vi "Washer HCC Tool.vi"() -> ()   [LabVIEW 2009]
panel:
  in  "Backup Batch File":path=path "c:/Program Files/GE/Washer HCC/robocopy_update.bat"
  out "COM Port":string
  in  "Station":u16(ring) items=["1", "2", "3", "4", "5", "6", "7", "8", "9", "10", "11", "12", "13", "14", "15", "16", "17", "18", "19", "20"]
  in  "Row":u16(ring) items=["A", "B", "C", "D", "E", "F", "G", "H", "I", "J", "M", "N", "S"]
  in  "Save Now":bool
  out "Filename":string
  out "Min to AutoSave":dbl format="%#_3g"
  in  "AutoSave Period(min)":dbl=60.0
  in  "Serial":string="E15"
  in  "Unit":string="asssdf"
  out "date/time string":string
  in  "Station Com Unit Serial Array":string[][](array[string])
  in  "Clipboard":bool
  in  "OK":bool
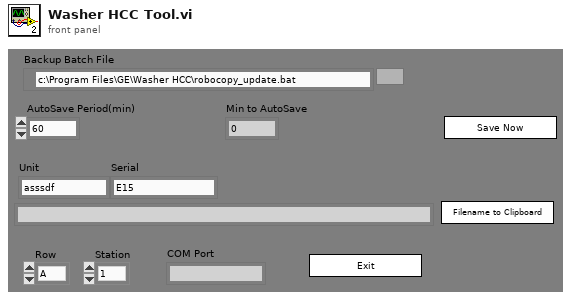
[diagram p1: front panel]
types:
  T1 = enum32{"invalid app kind", "Development System", "Run Time System", "Student Edition", "Embedded LabVIEW", "Evaluation", "Custom"}
  T2 = enum32{"Invalid", "Standard", "Closed", "Hidden", "Minimized", "Maximized"}
  T3 = cluster{"Core":cluster{"Current VI Reference":refnum<vi>, "Close Panel on Exit?":bool}, "Your Boolean data":bool, "Station Com Unit Serial Array":string[][], "Elapsed Time (sec)":dbl}
  T4 = cluster{"Current VI Reference":refnum<vi>, "Close Panel on Exit?":bool}
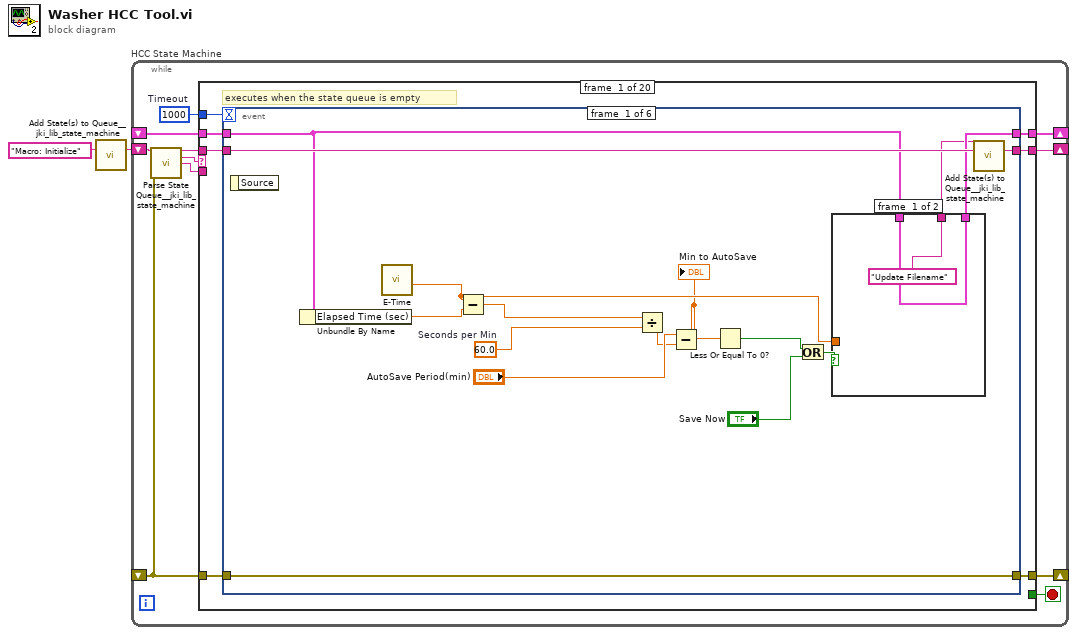
[diagram p0: block diagram]
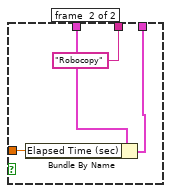
[diagram p2: hidden frame]
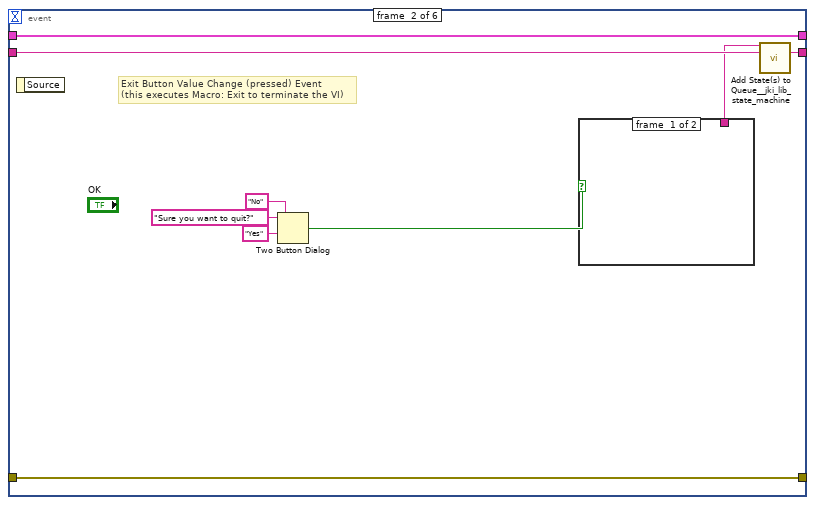
[diagram p3: hidden frame]
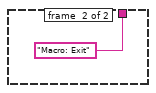
[diagram p4: hidden frame]
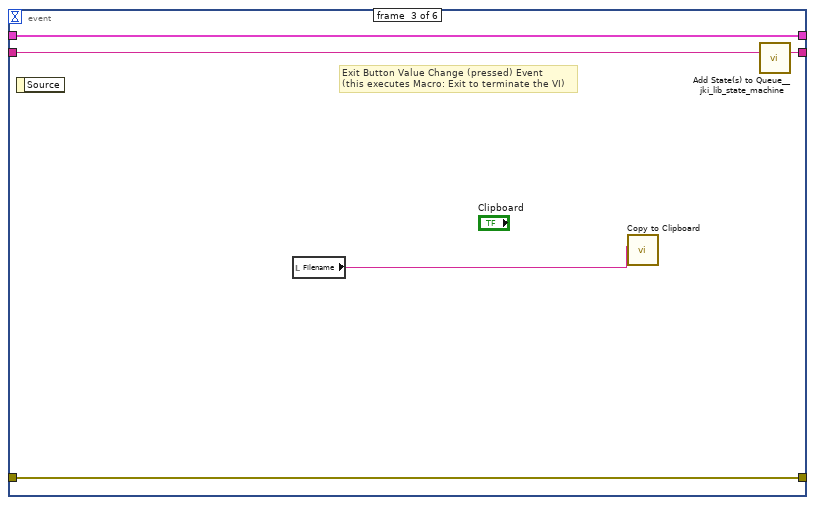
[diagram p5: hidden frame]
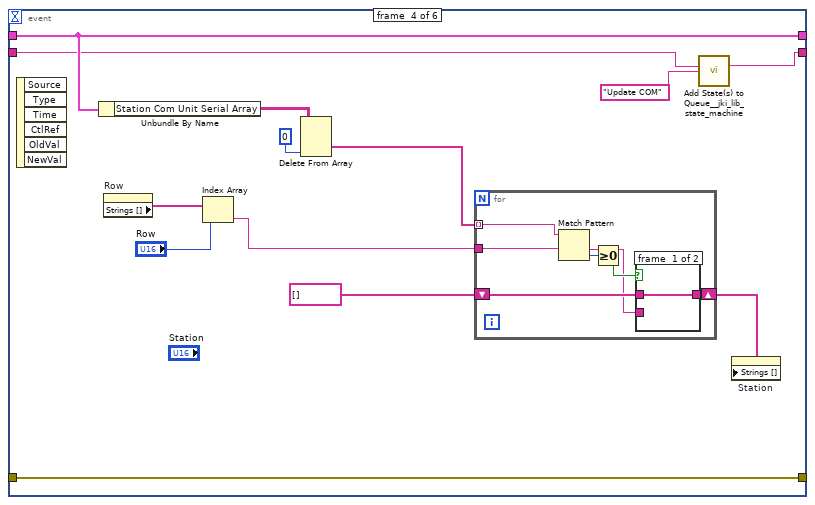
[diagram p6: hidden frame]
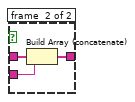
[diagram p7: hidden frame]
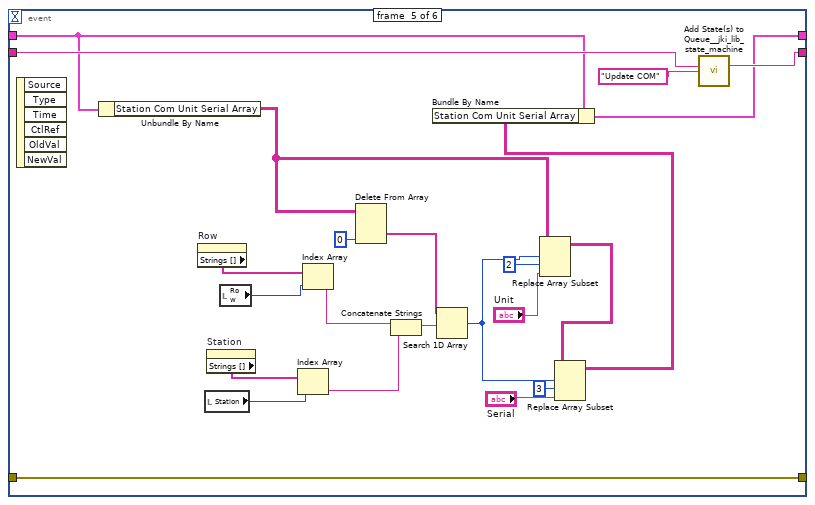
[diagram p8: hidden frame]
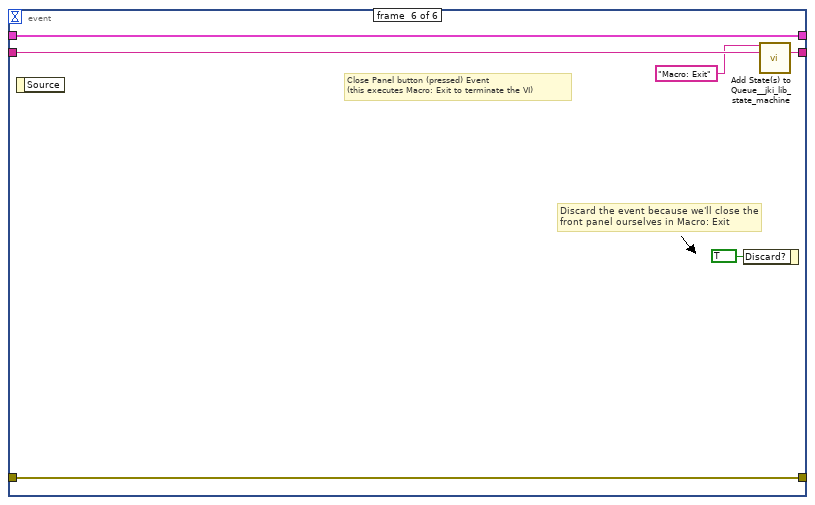
[diagram p9: hidden frame]
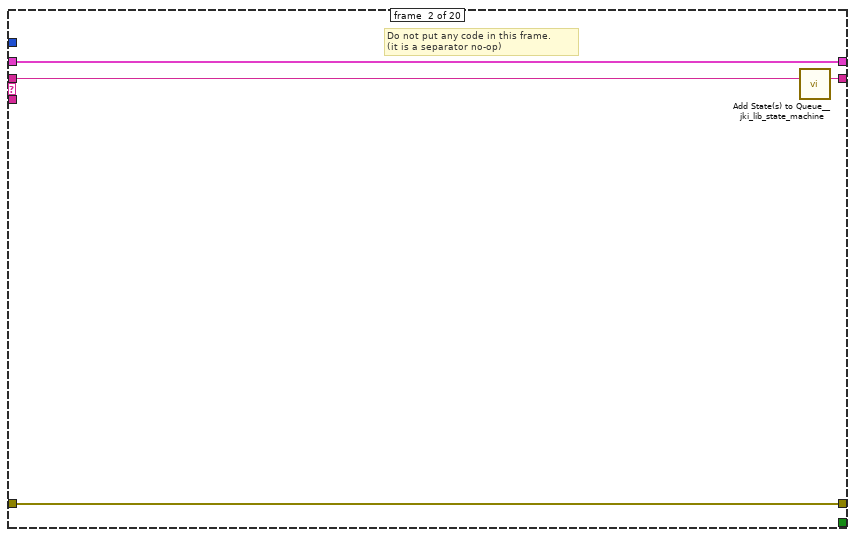
[diagram p10: hidden frame]
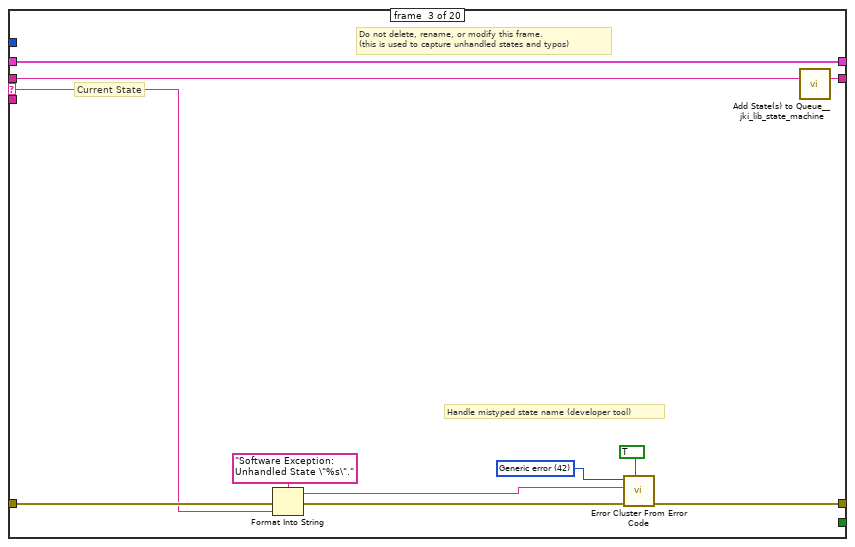
[diagram p11: hidden frame]
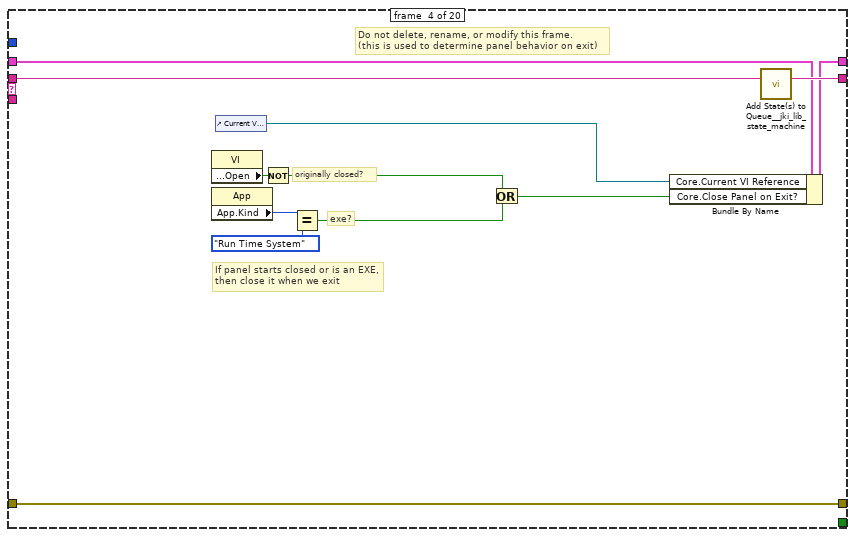
[diagram p12: hidden frame]
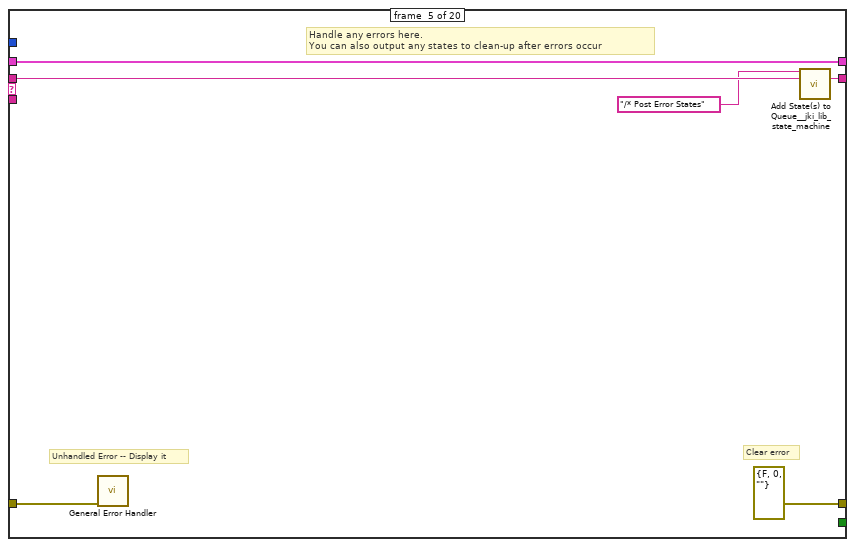
[diagram p13: hidden frame]
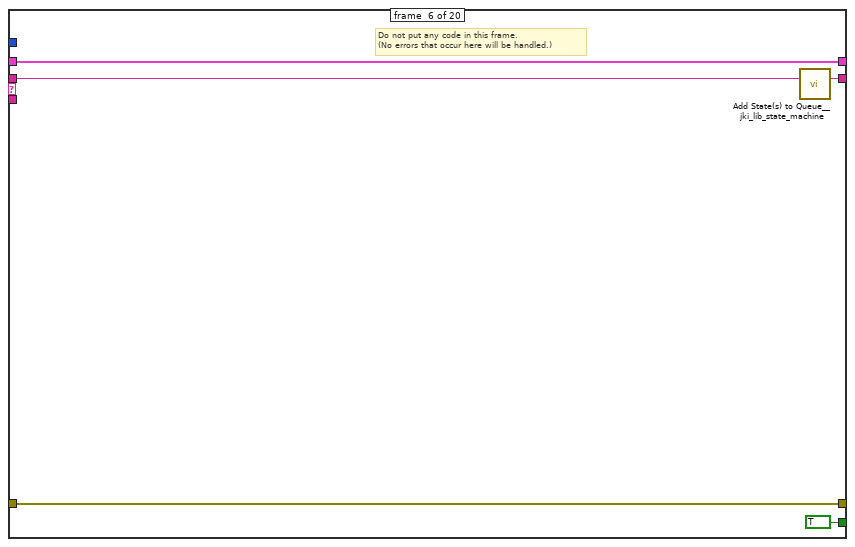
[diagram p14: hidden frame]
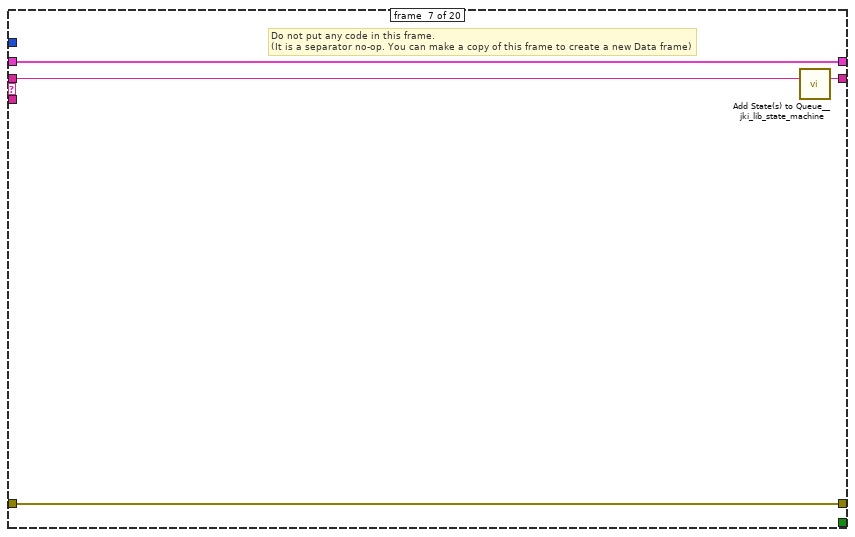
[diagram p15: hidden frame]
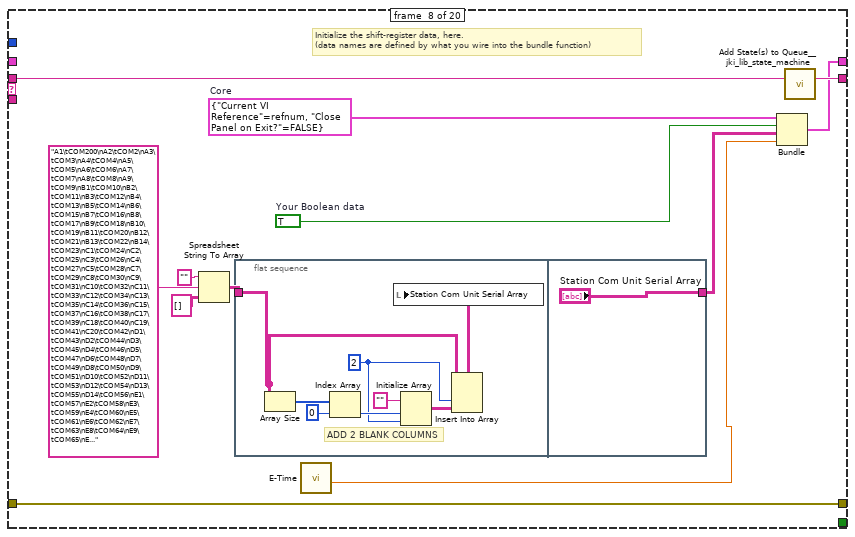
[diagram p16: hidden frame]
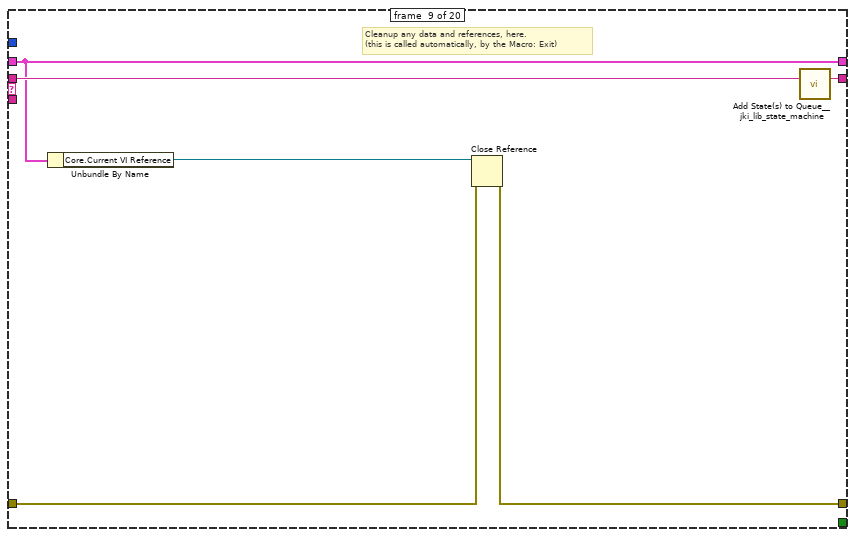
[diagram p17: hidden frame]
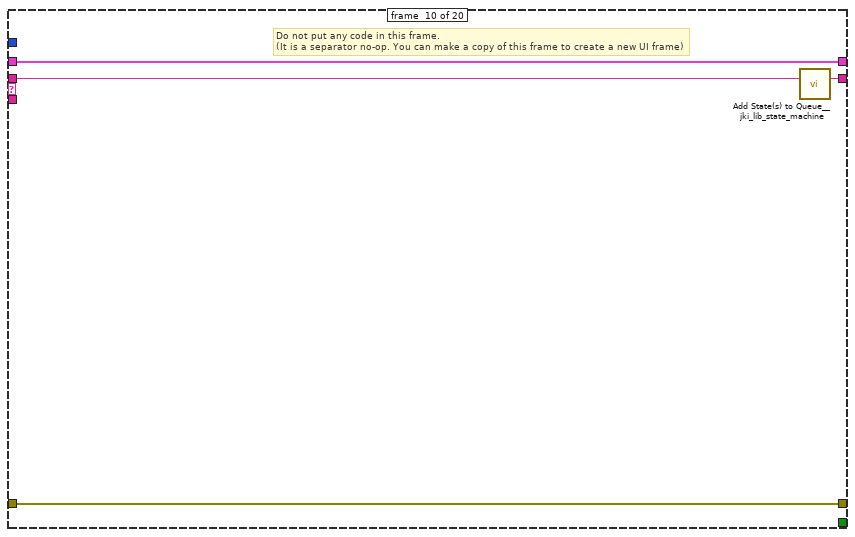
[diagram p18: hidden frame]
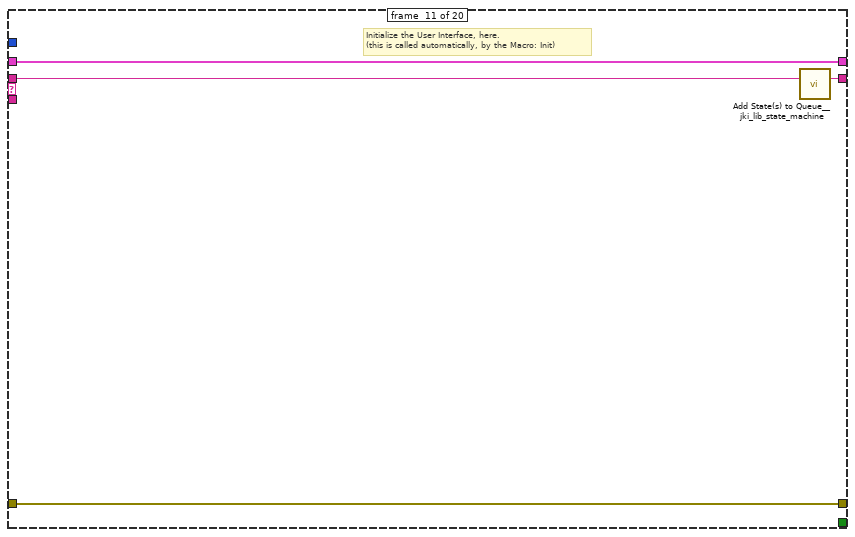
[diagram p19: hidden frame]
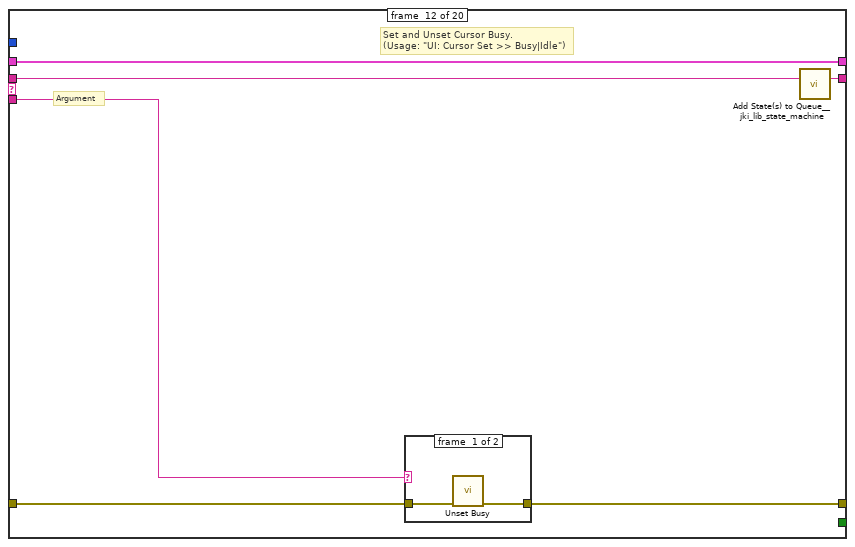
[diagram p20: hidden frame]
diagram:
  n1 = call <vilib>:"Add State(s) to Queue__jki_lib_state_machine.vi"("State(s) in (\"\")"="Macro: Initialize") -> ("States Out"=w2:string)  [unwired: 14 in]
  n2 = while "HCC State Machine" {
    shift-right: [w6] -> _
    shift-left: _ -> [w5]
    shift-right: [w9] -> _
    shift-left: _ -> [w3]
    shift-right: [w8] -> _
    shift-left: w2 -> [w10]
    stop <- w7 stop-if-true
    w4 = 1000  # Timeout
    n3 = call <vilib>:"Parse State Queue__jki_lib_state_machine.vi"("State Queue"=w10, "Error In (no error)"=w3) -> ("Remaining States"=w12:string, "Current State"=w13:string, "Arguments"=w11:string)  [unwired: 11 in]
    n4 = case shown="\"Data: Cleanup\"" w13 {
      selector: w13 -> [_ _ w115 _ _ _ _ _ _ _ _ _ _ _ _ _ _ _ _ _]
      tunnel: w12 -> [w20 w114 w119 w137 w143 w148 w152 w164 w179 w183 w187 w193 w204 w230 w235 w245 w249 w269 w276 w300]
      tunnel: w11 -> [_ _ _ _ _ _ _ _ _ _ _ w188 w198 _ _ _ _ _ _ _]
      tunnel: w5 -> [w18 w111 w117 w128 w140 w146 w149 _ w174 w180 w185 w191 w200 w227 w232 w242 w246 w266 w274 w297]
      tunnel: [w17 w112 w121 w134 errorcluster {"status"=FALSE, "code"=0, "source"=""} ("error out") w145 w150 w161 w175 w181 w184 w189 w201 w228 w233 w243 w247 w267 w272 w298] -> w9
      tunnel: w3 -> [w16 w112 w120 w134 w139 w145 w150 w161 w176 w181 w184 w190 w202 w228 w233 w243 w247 w267 w273 w298]
      tunnel: [w19 w113 w118 w136 w142 w147 w151 w163 w178 w182 w186 w192 w203 w229 w234 w244 w248 w268 w275 w299] -> w8
      tunnel: [_ _ _ _ _ TRUE _ _ _ _ _ _ _ _ _ _ _ _ _ _] -> w7
      tunnel: [w15 w111 w117 w135 w140 w146 w149 w162 w174 w180 w185 w191 w200 w227 w232 w242 w246 w266 w274 w297] -> w6
      tunnel: w4 -> [w14 _ _ _ _ _ _ _ _ _ _ _ _ _ _ _ _ _ _ _]
      frame #0 {
        # "executes when the state queue is empty"
        n5 = event shown="[4] \"Unit\", \"Serial\": Value Change" {
          selector: _ -> [_ _ _ _ _ _]
          dyn-events: _ -> [_ _ _ _ _ _]
          timeout: w14 -> [_ _ _ _ _ _]
          tunnel: w20 -> [w36 w51 w57 w60 w103 w110]
          tunnel: [w35 w50 w56 w59 w102 w109] -> w19
          tunnel: w18 -> [w28 w48 w54 w70 w90 w107]
          tunnel: [w34 w49 w55 w69 w104 w108] -> w17
          tunnel: w16 -> [w34 w49 w55 w69 w104 w108]
          tunnel: [w27 w48 w54 w70 w91 w107] -> w15
          event #0 {
            w31 = 60.0  # Seconds per Min
            n6 = event-data() -> ()  [unwired: 1 in, 1 out]
            n7 = Unbundle By Name(w28) -> ("Elapsed Time (sec)"=w33:dbl)
            n8 = call "E-Time.vi"() -> ("Elapsed Time (sec)"=w26:dbl)  [unwired: 9 in, 2 out]
            n9 = Subtract(x=w26, y=w33) -> (x-y=w32:dbl)
            n10 = Divide(x=w32, y=w31) -> (x/y=w22:dbl)
            n11 = Subtract(x="AutoSave Period(min)", y=w22) -> (x-y=w24:dbl)
            "Min to AutoSave" <- w24
            n12 = Less Or Equal To 0?(x=w24) -> (x <= 0?=w30:bool)
            n13 = Or(x=w30, y="Save Now") -> (x .or. y?=w29:bool)
            n14 = case shown="False" w29 {
              tunnel: w28 -> [w38 w41]
              tunnel: [w38 w42] -> w27
              tunnel: w26 -> [_ w40]
              tunnel: ["Update Filename" ("State(s) in Front (\"\")") "Robocopy" ("State(s) in Front (\"\")")] -> w25
              frame #0 {
              }
              frame #1 {
                n15 = Bundle By Name(cluster=w41, "Elapsed Time (sec)"=w40) -> (w42:T3)
              }
            }
            n16 = call <vilib>:"Add State(s) to Queue__jki_lib_state_machine.vi"("State(s) in Front (\"\")"=w25, "State(s) in (\"\")"=w36) -> ("States Out"=w35:string)  [unwired: 13 in]
          }
          event #1 {
            # "Exit Button Value Change (pressed) Event\n(this executes Macro: Exit to terminate the VI)"
            n17 = event-data() -> ()  [unwired: 1 in, 1 out]
            n18 = Two Button Dialog(message="Sure you want to quit?", 1:"No" ("F button name (\"Cancel\")"), 2:"Yes" ("T button name (\"OK\")")) -> (T button?=w43:bool)
            n19 = case shown="True" w43 {
              tunnel: [_ "Macro: Exit"] -> w47
              frame #0 {
              }
              frame #1 {
              }
            }
            n20 = call <vilib>:"Add State(s) to Queue__jki_lib_state_machine.vi"("State(s) in Front (\"\")"=w47, "State(s) in (\"\")"=w51) -> ("States Out"=w50:string)  [unwired: 13 in]
          }
          event #2 {
            # "Exit Button Value Change (pressed) Event\n(this executes Macro: Exit to terminate the VI)"
            n21 = event-data() -> ()  [unwired: 1 in, 1 out]
            n22 = local read "Filename"() -> (w53:string)
            n23 = call "Copy to Clipboard.vi"("Text"=w53) -> ()  [unwired: 11 in]
            n24 = call <vilib>:"Add State(s) to Queue__jki_lib_state_machine.vi"("State(s) in (\"\")"=w57) -> ("States Out"=w56:string)  [unwired: 14 in]
          }
          event #3 {
            n25 = event-data() -> ()  [unwired: 1 in, 6 out]
            n26 = Unbundle By Name(w70) -> ("Station Com Unit Serial Array"=w66:string[][])
            n27 = property on="Row" class="Ring (strict)"() -> ("Strings []"=w68:string[])  [unwired: 2 in, 2 out]
            n28 = Index Array(array=w68, index="Row") -> (element=w63:string)
            n29 = Delete From Array(array=w66, index (col)=0 ("length")) -> (deleted portion=w65:string[])  [unwired: 2 in, 1 out]
            n30 = for {
              tunnel: w65 -> [w77] mode=indexing
              tunnel: w63 -> [w76]
              shift-right: [w73] -> w61
              shift-left: string[] [] ("deleted portion") -> [w72]
              n31 = Match Pattern(string=w77, regular expression=w76) -> (after substring=w71:string, offset past match=w75:i32)  [unwired: 1 in, 2 out]
              n32 = Greater Or Equal To 0?(x=w75) -> (x >= 0?=w74:bool)
              n33 = case shown="True" w74 {
                tunnel: [w78 w80] -> w73
                tunnel: w72 -> [w78 w81]
                tunnel: w71 -> [_ w79]
                frame #0 {
                }
                frame #1 {
                  n34 = Build Array (concatenate)(w81, w79) -> (w80:string[])
                }
              }
            }
            n35 = call <vilib>:"Add State(s) to Queue__jki_lib_state_machine.vi"("State(s) in (\"\")"=w60, "State(s) at Back (\"\")"="Update COM" ("State(s) at Back (\"\")")) -> ("States Out"=w59:string)  [unwired: 13 in]
            n36 = property on="Station" class="Ring (strict)"("Strings []"=w61) -> ()  [unwired: 2 in, 2 out]
          }
          event #4 {
            n37 = event-data() -> ()  [unwired: 1 in, 6 out]
            n38 = Unbundle By Name(w90) -> ("Station Com Unit Serial Array"=w89:string[][])
            n39 = property on="Row" class="Ring (strict)"() -> ("Strings []"=w100:string[])  [unwired: 2 in, 2 out]
            n40 = local read "Station"() -> (w97:u16)
            n41 = property on="Station" class="Ring (strict)"() -> ("Strings []"=w98:string[])  [unwired: 2 in, 2 out]
            n42 = local read "Row"() -> (w99:u16)
            n43 = Index Array(array=w98, index=w97) -> (element=w95:string)
            n44 = Index Array(array=w100, index=w99) -> (element=w96:string)
            n45 = Delete From Array(array=w89, index (col)=0 ("disabled index (col)")) -> (deleted portion=w92:string[])  [unwired: 2 in, 1 out]
            n46 = Concatenate Strings(w96, w95) -> (w94:string)
            n47 = Search 1D Array(1D array=w92, element=w94) -> (index of element=w84:i32)  [unwired: 1 in]
            n48 = Replace Array Subset(array=w89, new element="Unit", index (row)=w84, index (col)=2 ("disabled index (col)")) -> (w86:string[][])
            n49 = Replace Array Subset(array=w86, new element="Serial", index (row)=w84, index (col)=3 ("disabled index (col)")) -> (w82:string[][])
            n50 = Bundle By Name(cluster=w90, "Station Com Unit Serial Array"=w82) -> (w91:T3)
            n51 = call <vilib>:"Add State(s) to Queue__jki_lib_state_machine.vi"("State(s) in (\"\")"=w103, "State(s) at Back (\"\")"="Update COM" ("State(s) at Back (\"\")")) -> ("States Out"=w102:string)  [unwired: 13 in]
          }
          event #5 {
            # "Discard the event because we'll close the front panel ourselves in Macro: Exit"
            # "Close Panel button (pressed) Event\n(this executes Macro: Exit to terminate the VI)"
            n52 = event-data() -> ()  [unwired: 1 in, 1 out]
            n53 = event-data("Discard?"=TRUE) -> ()  [unwired: 1 in, 1 out]
            n54 = call <vilib>:"Add State(s) to Queue__jki_lib_state_machine.vi"("State(s) in Front (\"\")"="Macro: Exit", "State(s) in (\"\")"=w110) -> ("States Out"=w109:string)  [unwired: 13 in]
          }
        }
      }
      frame #1 {
        # "Do not put any code in this frame.\n(it is a separator no-op)"
        n55 = call <vilib>:"Add State(s) to Queue__jki_lib_state_machine.vi"("State(s) in (\"\")"=w114) -> ("States Out"=w113:string)  [unwired: 14 in]
      }
      frame #2 {
        w124 = 42 items=["No error", "Argument error", "Memory is full", "Out of zone", "End of file", "File already open", "Generic file I/O error", "File not found", "File permission error", "Disk is full", "Duplicate path", "Too many files open", "System feature not enabled", "Resource file not found", "Cannot add resource", "Resource not found", "Image not found", "Image memory error", "Pen does not exist", "Config type invalid", "Config token not found", "Config parse error", "Config memory error", "Bad external code format", "Bad external code offset", "External code not present", "Null window", "Destroy window error", "Null menu", "Print aborted", "Bad print record", "Print driver error", "Windows error during printing", "Memory error during printing", "Print dialog error", "Generic print error", "Invalid device refnum", "Device not found", "Device parameter error", "Device unit error", "Cannot open device", "Device call aborted", "Generic error", "Cancelled by user", "Object ID too low", "Object ID too high", "Object not in heap", "Unknown heap", "Unknown object (invalid DefProc)", "Unknown object (DefProc not in table)", "Message out of range", "Invalid (null) method", "Unknown message", "Manager call not supported", "Bad address", "Network operation in progress", "Network operation timed out", "Connection is busy", "Network attribute not supported", "Network error", "Address in use", "System out of memory", "Connection aborted", "Connection refused", "Not connected", "Already connected", "Connection closed", "Initialization error (interapplication manager)", "Bad occurrence", "Wait on unbound occurrence handler", "Occurrence queue overflow", "Datalog type conflict", "Unused", "Unrecognized type (interapplication manager)", "Memory corrupt", "Failed to make temporary DLL", "Old CIN version", "Drag socket not found", "Failed to load drop-object", "Failed to register OLE object", "Failed to release OLE object", "Format specifier type mismatch", "Unknown format specifier", "Too few format specifiers", "Too many format specifiers", "Scan failed", "Newer CIN version", "Error converting to variant", "Runtime menu error", "Password tampered", "Variant attribute not found", "Incompatible variant data type", "Event data is not available", "Event Store is not present", "Occurrence is not found", "Event Queue is not created", "Event info is not available", "Refnum passed is NULL", "Error retrieving Class GUID", "Error retrieving CoClass GUID", "Error retrieving TypeLib GUID.", "Bad built application magic bytes.", "Specific driver is different from the specific driver associated with the Logical Name.", "There is no session opened to the class driver.", "Max Error", "MAX - Error with config objects", "MAX - Error loading configuration", "MAX - Group not supported"]
        # "Current State"
        # "Do not delete, rename, or modify this frame.\n(this is used to capture unhandled states and typos)"
        # "Handle mistyped state name (developer tool)"
        n56 = Format Into String(format string="Software Exception: Unhandled State \"%s\"." ("message"), error in=w120, w115) -> (resulting string=w123:string, error out=w122:errorcluster)  [unwired: 1 in]
        n57 = call <vilib>:"Error Cluster From Error Code.vi"("show call chain? (False)"=TRUE, "error in (no error)"=w122, "error message (\"\")"=w123, "error code (0)"=w124) -> ("error out"=w121:errorcluster)  [unwired: 5 in]
        n58 = call <vilib>:"Add State(s) to Queue__jki_lib_state_machine.vi"("State(s) in (\"\")"=w119) -> ("States Out"=w118:string)  [unwired: 14 in]
      }
      frame #3 {
        # "Do not delete, rename, or modify this frame.\n(this is used to determine panel behavior on exit)"
        # "originally closed?"
        # "exe?"
        # "If panel starts closed or is an EXE, then close it when we exit"
        n59 = property class="VI"() -> ("Front Panel.Open"=w133:bool)  [unwired: 2 in, 2 out]
        n60 = property class="App"() -> ("App.Kind"=w132:T1)  [unwired: 2 in, 2 out]
        n61 = control-ref of="Current VI Reference"() -> (w126:refnum<vi>)
        n62 = Not(x=w133) -> (.not. x?=w130:bool)
        n63 = Equal?(x=w132, y=T1."Run Time System" ("Application:Kind")) -> (x = y?=w129:bool)
        n64 = Or(x=w130, y=w129) -> (x .or. y?=w127:bool)
        n65 = Bundle By Name(cluster=w128, "Core.Current VI Reference"=w126, "Core.Close Panel on Exit?"=w127) -> (w135:T3)
        n66 = call <vilib>:"Add State(s) to Queue__jki_lib_state_machine.vi"("State(s) in (\"\")"=w137) -> ("States Out"=w136:string)  [unwired: 14 in]
      }
      frame #4 {
        # "Unhandled Error -- Display it"
        # "Handle any errors here.\nYou can also output any states to clean-up after errors occur"
        # "Clear error"
        n67 = call <vilib>:"General Error Handler.vi"("error in (no error)"=w139) -> ()  [unwired: 10 in, 5 out]
        n68 = call <vilib>:"Add State(s) to Queue__jki_lib_state_machine.vi"("State(s) in Front (\"\")"="/* Post Error States", "State(s) in (\"\")"=w143) -> ("States Out"=w142:string)  [unwired: 13 in]
      }
      frame #5 {
        # "Do not put any code in this frame.\n(No errors that occur here will be handled.)"
        n69 = call <vilib>:"Add State(s) to Queue__jki_lib_state_machine.vi"("State(s) in (\"\")"=w148) -> ("States Out"=w147:string)  [unwired: 14 in]
      }
      frame #6 {
        # "Do not put any code in this frame.\n(It is a separator no-op. You can make a copy of this frame to create a new Data frame)"
        n70 = call <vilib>:"Add State(s) to Queue__jki_lib_state_machine.vi"("State(s) in (\"\")"=w152) -> ("States Out"=w151:string)  [unwired: 14 in]
      }
      frame #7 {
        w159 = T4 {"Current VI Reference"=refnum, "Close Panel on Exit?"=FALSE}  # Core
        w160 = TRUE  # Your Boolean data
        # "Initialize the shift-register data, here.\n(data names are defined by what you wire into the bundle function)"
        n71 = Spreadsheet String To Array(format string="", spreadsheet string="A1\tCOM200\nA2\tCOM2\nA3\tCOM3\nA4\tCOM4\nA5\tCOM5\nA6\tCOM6\nA7\tCOM7\nA8\tCOM8\nA9\tCOM9\nB1\tCOM10\nB2\tCOM11\nB3\tCOM12\nB4\tCOM13\nB5\tCOM14\nB6\tCOM15\nB7\tCOM16\nB8\tCOM17\nB9\tCOM18\nB10\tCOM19\nB11\tCOM20\nB12\tCOM21\nB13\tCOM22\nB14\tCOM23\nC1\tCOM24\nC2\tCOM25\nC3\tCOM26\nC4\tCOM27\nC5\tCOM28\nC7\tCOM29\nC8\tCOM30\nC9\tCOM31\nC10\tCOM32\nC11\tCOM33\nC12\tCOM34\nC13\tCOM35\nC14\tCOM36\nC15\tCOM37\nC16\tCOM38\nC17\tCOM39\nC18\tCOM40\nC19\tCOM41\nC20\tCOM42\nD1\tCOM43\nD2\tCOM44\nD3\tCOM45\nD4\tCOM46\nD5\tCOM47\nD6\tCOM48\nD7\tCOM49\nD8\tCOM50\nD9\tCOM51\nD10\tCOM52\nD11\tCOM53\nD12\tCOM54\nD13\tCOM55\nD14\tCOM56\nE1\tCOM57\nE2\tCOM58\nE3\tCOM59\nE4\tCOM60\nE5\tCOM61\nE6\tCOM62\nE7\tCOM63\nE8\tCOM64\nE9\tCOM65\nE10\tCOM66\nE11\tCOM67\nE12\tCOM68\nE13\tCOM69\nE14\tCOM70\nE15\tCOM71\nE16\tCOM72\nE17\tCOM73\nE18\tCOM74\nE19\tCOM75\nE20\tCOM76\nF1\tCOM77\nF2\tCOM78\nF5\tCOM79\nF6\tCOM80\nF7\tCOM81\nF8\tCOM82\nF9\tCOM83\nF10\tCOM84\nF11\tCOM85\nF12\tCOM86\nF13\tCOM87\nG1\tCOM88\nG2\tCOM89\nG3\tCOM90\nG4\tCOM91\nG5\tCOM92\nG6\tCOM93\nG7\tCOM94\nG8\tCOM95\nG9\tCOM96\nG10\tCOM97\nG11\tCOM98\nG12\tCOM99\nG13\tCOM100\nG14\tCOM101\nH1\tCOM102\nH2\tCOM103\nH3\tCOM104\nH4\tCOM105\nH5\tCOM106\nH6\tCOM107\nH7\tCOM108\nH8\tCOM109\nH9\tCOM110\nH10\tCOM111\nI1\tCOM112\nI2\tCOM113\nI3\tCOM114\nI4\tCOM115\nI5\tCOM116\nI6\tCOM117\nI7\tCOM118\nI8\tCOM119\nI9\tCOM120\nI10\tCOM121\nI11\tCOM122\nI12\tCOM123\nM1\tCOM100\nM2\tCOM2\nM3\tCOM3\nM4\tCOM4\nM5\tCOM5\nM6\tCOM6\nM7\tCOM7\nM8\tCOM8\nM9\tCOM9\nM10\tCOM10\nM11\tCOM11\nM12\tCOM12\nM13\tCOM13\nM14\tCOM14\nM15\tCOM15\nM16\tCOM16\nM17\tCOM17\nM18\tCOM18\nM19\tCOM19\nM20\tCOM20\nN6\tCOM21\nN7\tCOM22\nN8\tCOM23\nN9\tCOM24\nN10\tCOM25\nN11\tCOM26\nN12\tCOM27\nN13\tCOM28\nS1\tCOM29\nS2\tCOM30\nS3\tCOM31\nS4\tCOM32\nS5\tCOM33\nS6\tCOM34\nS7\tCOM35\nS8\tCOM36\nS9\tCOM37\nS10\tCOM38\nS11\tCOM39\nS12\tCOM40\nS13\tCOM41\nS14\tCOM42\nS15\tCOM43\nS16\tCOM44\nS17\tCOM45\nS18\tCOM46\nS19\tCOM47\nS20\tCOM48\n", array type (2D Dbl)=string[][] []) -> (array=w154:string[][])  [unwired: 1 in]
        n72 = flat-sequence {
          tunnel: w154 -> [w166]
          tunnel: ["Station Com Unit Serial Array"] -> w157
          frame #0 {
            w169 = 2 ("index (row)")
            # "ADD 2 BLANK COLUMNS"
            n73 = Array Size(array=w166) -> (size(s)=w172:i32[])
            n74 = Index Array(array=w172, index=0) -> (element=w170:i32)
            n75 = Initialize Array("", w170, w169) -> (w167:string[][])
            n76 = Insert Into Array(array=w166, index (col)=w169, new element=w167) -> (w165:string[][])  [unwired: 1 in]
            n77 = local write "Station Com Unit Serial Array"(w165) -> ()
          }
          frame #1 {
          }
        }
        n78 = call "E-Time.vi"() -> ("Elapsed Time (sec)"=w153:dbl)  [unwired: 9 in, 2 out]
        n79 = Bundle("Core"=w159, "Your Boolean data"=w160, "Station Com Unit Serial Array"=w157, "Elapsed Time (sec)"=w153) -> (w162:T3)  [unwired: 1 in]
        n80 = call <vilib>:"Add State(s) to Queue__jki_lib_state_machine.vi"("State(s) in (\"\")"=w164) -> ("States Out"=w163:string)  [unwired: 14 in]
      }
      frame #8 {
        # "Cleanup any data and references, here.\n(this is called automatically, by the Macro: Exit)"
        n81 = Unbundle By Name(w174) -> ("Core.Current VI Reference"=w177:refnum<vi>)
        n82 = Close Reference(reference=w177, error in (no error)=w176) -> (error out=w175:errorcluster)
        n83 = call <vilib>:"Add State(s) to Queue__jki_lib_state_machine.vi"("State(s) in (\"\")"=w179) -> ("States Out"=w178:string)  [unwired: 14 in]
      }
      frame #9 {
        # "Do not put any code in this frame.\n(It is a separator no-op. You can make a copy of this frame to create a new UI frame)"
        n84 = call <vilib>:"Add State(s) to Queue__jki_lib_state_machine.vi"("State(s) in (\"\")"=w183) -> ("States Out"=w182:string)  [unwired: 14 in]
      }
      frame #10 {
        # "Initialize the User Interface, here.\n(this is called automatically, by the Macro: Init)"
        n85 = call <vilib>:"Add State(s) to Queue__jki_lib_state_machine.vi"("State(s) in (\"\")"=w187) -> ("States Out"=w186:string)  [unwired: 14 in]
      }
      frame #11 {
        # "Argument"
        # "Set and Unset Cursor Busy.\n(Usage: \"UI: Cursor Set >> Busy|Idle\")"
        n86 = case shown="\"Idle\", Default" w188 {
          tunnel: w190 -> [w195 w197]
          tunnel: [w194 w196] -> w189
          frame #0 {
            n87 = call <vilib>:"Unset Busy.vi"("error in (no error)"=w195) -> ("error out"=w194:errorcluster)  [unwired: 10 in]
          }
          frame #1 {
            n88 = call <vilib>:"Set Busy.vi"("error in (no error)"=w197) -> ("error out"=w196:errorcluster)  [unwired: 9 in, 1 out]
          }
        }
        n89 = call <vilib>:"Add State(s) to Queue__jki_lib_state_machine.vi"("State(s) in (\"\")"=w193) -> ("States Out"=w192:string)  [unwired: 14 in]
      }
      frame #12 {
        # "Argument"
        # "Set Front Panel Open or Closed\n(Usage: \"UI: Front Panel State >> Open|Close\")"
        n90 = Unbundle By Name(w200) -> ("Core.Current VI Reference"=w199:refnum<vi>)
        n91 = case shown="\"Open\", Default" w198 {
          tunnel: w202 -> [w208 w221]
          tunnel: [w210 w222] -> w201
          tunnel: w199 -> [w209 w219]
          frame #0 {
            n92 = property class="VI"(reference=w209, error in=w208) -> (reference out=w206:refnum<vi>, error out=w207:errorcluster, "Front Panel.Open"=w205:bool)
            n93 = case shown="False" w205 {
              tunnel: [w213 w216] -> w210
              tunnel: w207 -> [w212 w216]
              tunnel: w206 -> [w211 _]
              frame #0 {
                n94 = invoke class="VI" method="FP.Open"(reference=w211, error in=w212, "Activate"=TRUE, "State"=T2."Standard") -> (error out=w213:errorcluster)  [unwired: 1 in, 4 out]
              }
              frame #1 {
              }
            }
          }
          frame #1 {
            n95 = property class="VI"(reference=w219, error in=w221) -> (reference out=w218:refnum<vi>, error out=w220:errorcluster, "Front Panel.Open"=w217:bool)
            n96 = case shown="True" w217 {
              tunnel: [w223 w226] -> w222
              tunnel: w220 -> [w223 w225]
              tunnel: w218 -> [_ w224]
              frame #0 {
              }
              frame #1 {
                n97 = invoke class="VI" method="FP.Close"(reference=w224, error in=w225) -> (error out=w226:errorcluster)  [unwired: 1 in, 2 out]
              }
            }
          }
        }
        n98 = call <vilib>:"Add State(s) to Queue__jki_lib_state_machine.vi"("State(s) in (\"\")"=w204) -> ("States Out"=w203:string)  [unwired: 14 in]
      }
      frame #13 {
        # "Do not put any code in this frame.\n(It is a separator no-op. You can make a copy of this frame to create a new Macro frame)"
        n99 = call <vilib>:"Add State(s) to Queue__jki_lib_state_machine.vi"("State(s) in (\"\")"=w230) -> ("States Out"=w229:string)  [unwired: 14 in]
      }
      frame #14 {
        w231 = "Data: Initialize\nInitialize Core Data\nUI: Initialize\nUI: Front Panel State >> Open"  # Data: Initialize Initialize Core Data UI: Initialize UI: Front Panel State >> Open
        # "Initialization Macro\n(This is called once, when the VI starts)"
        n100 = call <vilib>:"Add State(s) to Queue__jki_lib_state_machine.vi"("State(s) in Front (\"\")"=w231, "State(s) in (\"\")"=w235) -> ("States Out"=w234:string)  [unwired: 13 in]
      }
      frame #15 {
        # "Exit Macro\n(This is called once, when the VI exits)"
        n101 = Unbundle By Name(w242) -> ("Core.Close Panel on Exit?"=w241:bool)
        n102 = Select(t="UI: Front Panel State >> Close", s=w241, f="") -> (s? t:f=w238:string)
        n103 = call <vilib>:"Add State(s) to Queue__jki_lib_state_machine.vi"("State(s) in (\"\")"=w238, "State(s) at Back (\"\")"="Data: Cleanup\nExit") -> ("States Out"=w236:string)  [unwired: 13 in]
        n104 = call <vilib>:"Add State(s) to Queue__jki_lib_state_machine.vi"("State(s) in Front (\"\")"=w236, "State(s) in (\"\")"=w245) -> ("States Out"=w244:string)  [unwired: 13 in]
      }
      frame #16 {
        # "Template Separator\n(You can make a copy of, or modify, this frame)"
        n105 = call <vilib>:"Add State(s) to Queue__jki_lib_state_machine.vi"("State(s) in (\"\")"=w249) -> ("States Out"=w248:string)  [unwired: 14 in]
      }
      frame #17 {
        w262 = "_" ("string")
        # "Your code here.\n(You can make a copy of, or modify, this frame)"
        n106 = property on="Row" class="Ring (strict)"() -> ("Strings []"=w259:string[])  [unwired: 2 in, 2 out]
        n107 = local read "Station"() -> (w256:u16)
        n108 = property on="Station" class="Ring (strict)"() -> ("Strings []"=w257:string[])  [unwired: 2 in, 2 out]
        n109 = local read "Row"() -> (w258:u16)
        n110 = local read "Serial"() -> (w251:string)
        n111 = Index Array(array=w257, index=w256) -> (element=w260:string)
        n112 = local read "Unit"() -> (w250:string)
        n113 = Index Array(array=w259, index=w258) -> (element=w253:string)
        n114 = Format Date/Time String(time format string (%c)="%y%m%d_%H%M") -> (date/time string=w264:string)  [unwired: 2 in]
        "date/time string" <- w264
        n115 = Concatenate Strings(w253, w260) -> (w255:string)
        n116 = Concatenate Strings("D:\\Data\\HCC Debug Log Data\\Row " ("string"), w253, "\\" ("string"), w250, w262, w264, w262, w251, w262, w255, ".txt" ("string")) -> (→"Filename":string)
        n117 = call <vilib>:"Add State(s) to Queue__jki_lib_state_machine.vi"("State(s) in (\"\")"=w269) -> ("States Out"=w268:string)  [unwired: 14 in]
      }
      frame #18 {
        # "Your code here.\n(You can make a copy of, or modify, this frame)"
        n118 = Path To String(path="Backup Batch File") -> (string=w270:string)
        n119 = call <vilib>:"System Exec.vi"("error in (no error)"=w273, "command line"=w270) -> ("error out"=w272:errorcluster)  [unwired: 6 in, 3 out]
        n120 = call <vilib>:"Add State(s) to Queue__jki_lib_state_machine.vi"("State(s) in (\"\")"=w276) -> ("States Out"=w275:string)  [unwired: 14 in]
      }
      frame #19 {
        # "Your code here.\n(You can make a copy of, or modify, this frame)"
        n121 = Unbundle By Name(w297) -> ("Station Com Unit Serial Array"=w282:string[][])
        n122 = property on="Row" class="Ring (strict)"() -> ("Strings []"=w296:string[])  [unwired: 2 in, 2 out]
        n123 = local read "Station"() -> (w293:u16)
        n124 = property on="Station" class="Ring (strict)"() -> ("Strings []"=w294:string[])  [unwired: 2 in, 2 out]
        n125 = local read "Row"() -> (w295:u16)
        n126 = Index Array(array=w294, index=w293) -> (element=w291:string)
        n127 = Index Array(array=w296, index=w295) -> (element=w292:string)
        n128 = Delete From Array(array=w282, index (col)=0 ("disabled index (col)")) -> (deleted portion=w288:string[])  [unwired: 2 in, 1 out]
        n129 = Concatenate Strings(w292, w291) -> (w290:string)
        n130 = Search 1D Array(1D array=w288, element=w290) -> (index of element=w278:i32)  [unwired: 1 in]
        n131 = Delete From Array(array=w282, index (col)=1 ("disabled index (col)")) -> (deleted portion=w286:string[])  [unwired: 2 in, 1 out]
        n132 = Delete From Array(array=w282, index (col)=2 ("disabled index (col)")) -> (deleted portion=w280:string[])  [unwired: 2 in, 1 out]
        n133 = Delete From Array(array=w282, index (col)=3 ("disabled index (col)")) -> (deleted portion=w279:string[])  [unwired: 2 in, 1 out]
        n134 = Index Array(array=w286, index=w278) -> (element=→"COM Port":string)
        n135 = Index Array(array=w280, index=w278) -> (element=w281:string)
        n136 = Index Array(array=w279, index=w278) -> (element=w277:string)
        n137 = local write "Unit"(w281) -> ()
        n138 = local write "Serial"(w277) -> ()
        n139 = call <vilib>:"Add State(s) to Queue__jki_lib_state_machine.vi"("State(s) in (\"\")"=w300) -> ("States Out"=w299:string)  [unwired: 14 in]
      }
    }
  }
